vi "Read Parity Start Index.vi"(8 "error in (no error)":errorcluster, 11 "ARINC 429 in":refnum<class "ARINC 429.lvclass">) -> (0 "error out":errorcluster, 2 "parity start index":i32=31, 3 "ARINC 429 out":refnum<class "ARINC 429.lvclass">)   [LabVIEW 2020, in "ARINC 429.lvclass"]
uses:
  ARINC 429.lvclass
  ARINC 429.lvclass/ARINC 429.ctl
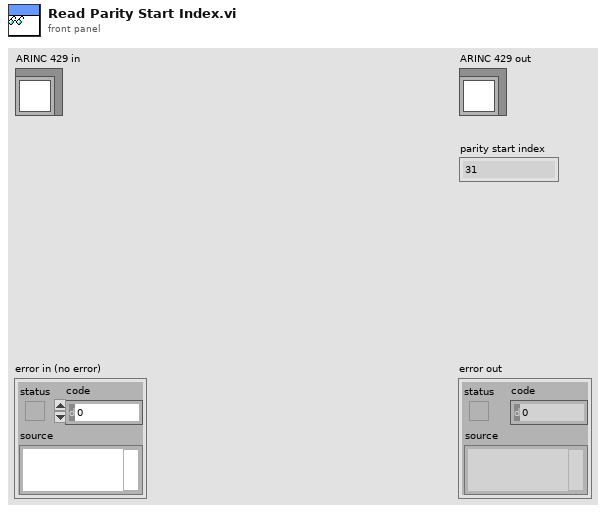
[diagram p1: front panel]
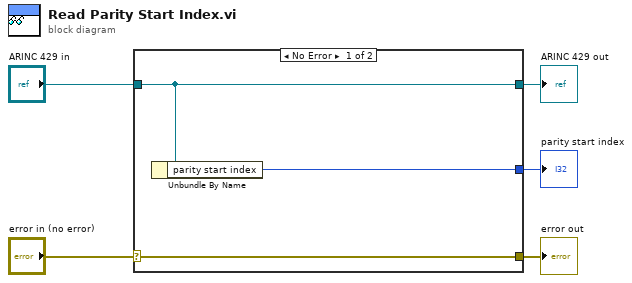
[diagram p0: block diagram]
diagram:
  n1 = case shown="No Error" "error in (no error)" {
    selector: "error in (no error)" -> [w8 w9]
    tunnel: [w8 w9] -> w4
    tunnel: [w7 w10] -> w2
    tunnel: "ARINC 429 in" -> [w7 w10]
    tunnel: [w6 _] -> w1
    frame No Error {
      n2 = Unbundle By Name(w7) -> ("parity start index"=w6:i32)
    }
    frame Error {
    }
  }
  "error out" <- w4
  "ARINC 429 out" <- w2
  "parity start index" <- w1
